vi "Initialize Serial Port.vi"(0 "VISA resource name":refnum<visa-resource-name>, 7 "baud rate (115200)":u32=115200, 11 "error in (no error)":errorcluster) -> (15 "error out":errorcluster)   [LabVIEW 2024, in "GRBL 1.1.lvlib"]
doc: "This VI initialise the serial port of the selected controller."
uses:
  GRBL 1.1.lvlib
  <vilib>/Instr/_visa.llb/VISA Configure Serial Port (Instr).vi
panel:
  out "String":string
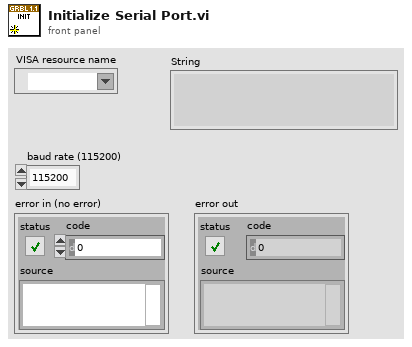
[diagram p1: front panel]
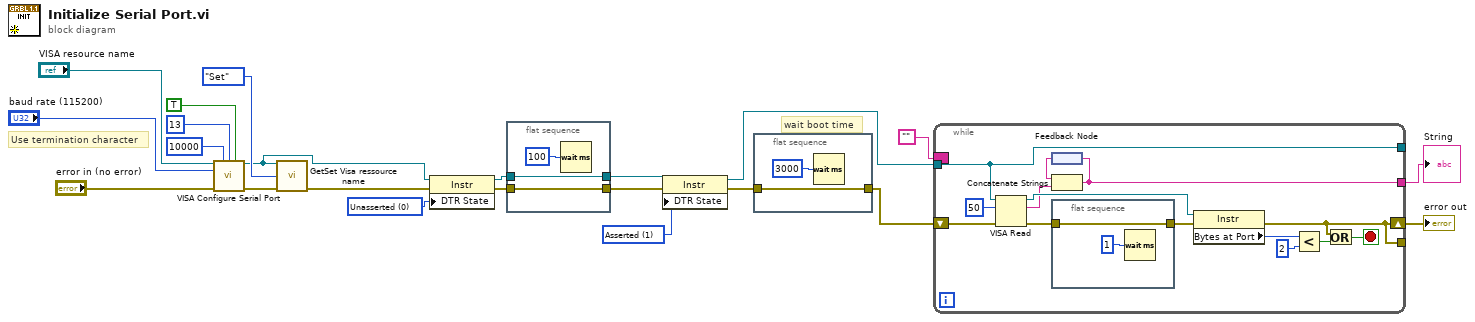
[diagram p0: block diagram]
diagram:
  w1 = i16 0 items=["Unknown"=-1, "Unasserted"=0, "Asserted"=1] ("Serial Settings:Modem Line Settings:Line DTR State")
  w2 = i16 1 items=["Unknown"=-1, "Unasserted"=0, "Asserted"=1] ("Serial Settings:Modem Line Settings:Line DTR State")
  # "Use termination character"
  # "wait boot time"
  n1 = call-poly "VISA Configure Serial Port"("VISA resource name"="VISA resource name", "timeout (10sec)"=u32 10000, "termination char\n(0xA = '\\n' = LF)"=u8 13 ("termination char\n(0xA = '\\n' = LF)"), "Enable Termination\nChar (T)"=TRUE ("Enable Termination\nChar (T)"), "baud rate (9600)"="baud rate (115200)", "error in (no error)"="error in (no error)") -> ("VISA resource name out"=w7:refnum<visa-resource-name>, "error out"=w20:errorcluster)  [unwired: 8 in]
  n2 = call "GetSet Visa ressource name.vi"("VISA resource name  in"=w7, "Get/Set"=enum16{"Get", "Set"}."Set", "error in (no error)"=w20) -> ("error out"=w16:errorcluster)  [unwired: 11 in, 1 out]
  n3 = property class="Instr"(reference=w7, error in=w16, "DTR State"=w1) -> (reference out=w5:refnum<visa-resource-name>, error out=w3:errorcluster)
  n4 = flat-sequence {
    tunnel: [w24] -> w6
    tunnel: w5 -> [w24]
    tunnel: [w23] -> w4
    tunnel: w3 -> [w23]
    frame #0 {
      n5 = Wait (ms)(milliseconds to wait=u32 100) -> ()  [unwired: 1 out]
    }
  }
  n6 = property class="Instr"(reference=w6, error in=w4, "DTR State"=w2) -> (reference out=w9:refnum<visa-resource-name>, error out=w13:errorcluster)
  n7 = flat-sequence {
    tunnel: w13 -> [w26]
    tunnel: [w26] -> w8
    frame #0 {
      n8 = Wait (ms)(milliseconds to wait=u32 3000) -> ()  [unwired: 1 out]
    }
  }
  n9 = while {
    tunnel: [w28] -> _
    tunnel: [w37] -> w10
    tunnel: [w33] -> _
    shift-right: [w33] -> w12
    shift-left: w8 -> [w41]
    border: "" -> [_]
    tunnel: w9 -> [w28]
    stop <- w34 stop-if-true
    n10 = VISA Read(VISA resource name=w28, byte count=u32 50, error in (no error)=w41) -> (VISA resource name out=w39:refnum<visa-resource-name>, read buffer=w32:string, error out=w31:errorcluster)  [unwired: 1 out]
    n11 = feedback #1() -> (w38:string)
    n12 = Concatenate Strings(w38, w32) -> (w37:string)
    n13 = feedback-in #1(w37) -> ()
    n14 = flat-sequence {
      tunnel: w31 -> [w42]
      tunnel: [w42] -> w30
      frame #0 {
        n15 = Wait (ms)(milliseconds to wait=u32 1) -> ()  [unwired: 1 out]
      }
    }
    n16 = property class="Instr"(reference=w39, error in=w30) -> (error out=w33:errorcluster, "Bytes at Port"=w29:u32)  [unwired: 1 out]
    n17 = Less?(x=w29, y=u32 2) -> (x < y?=w36:bool)
    n18 = Or(x=w33, y=w36) -> (x .or. y?=w34:bool)
  }
  "error out" <- w12
  "String" <- w10
